vi "Save Console Logs.vi"(0 "Barcode":string, 11 "Error In":errorcluster) -> (15 "Error Out":errorcluster)   [LabVIEW 2021]
doc: "Creates a text file and dumps the console logs into it."
uses:
  Controls/Console Manager Functions.ctl
panel:
  # "Inputs"
  # "Outputs"
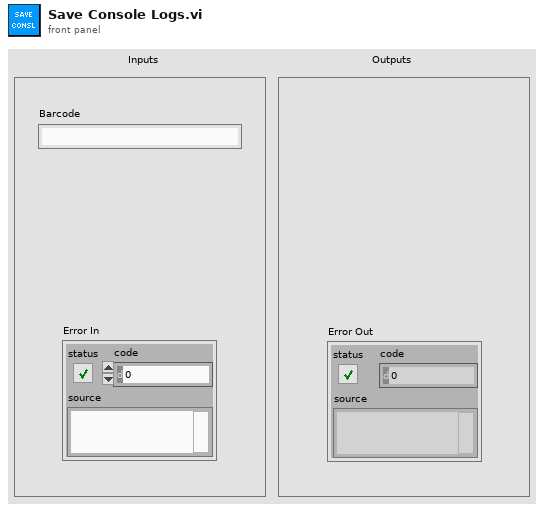
[diagram p1: front panel]
types:
  T1 = enum16{"open", "replace", "create", "open or create", "replace or create", "replace or create with confirmation"}
  T2 = typedef "Console Manager Functions.ctl" = enum16{"Init", "Add", "Get"}
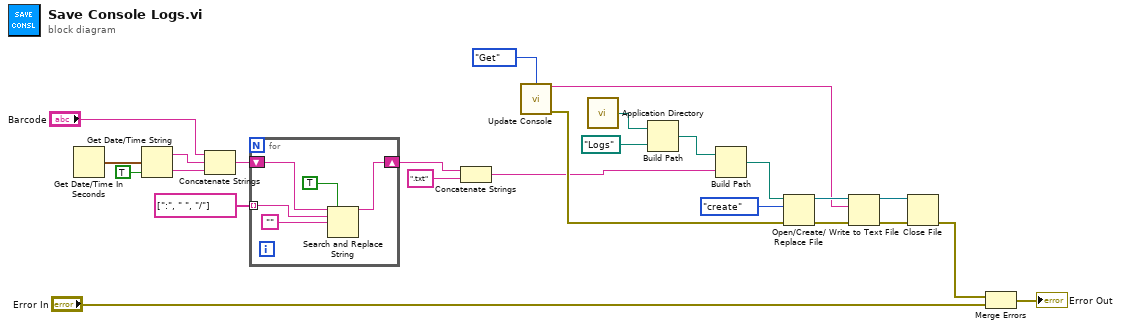
[diagram p0: block diagram]
diagram:
  n1 = Get Date/Time In Seconds() -> (seconds since 1Jan1904=w10:timestamp)
  n2 = Get Date/Time String(seconds (now)=w10, want seconds? (F)=TRUE) -> (date string=w7:string, time string=w8:string)  [unwired: 1 in]
  n3 = Concatenate Strings("Barcode", w7, w8) -> (w6:string)
  n4 = for {
    shift-right: [w27] -> w4
    shift-left: w6 -> [w29]
    tunnel: string[] [":", " ", "/"] ("search string") -> [w28] mode=indexing
    n5 = Search and Replace String(replace all?=TRUE ("replace all? (F)"), input string=w29, search string=w28, replace string="") -> (result string=w27:string)  [unwired: 4 in, 3 out]
  }
  n6 = Concatenate Strings(w4, ".txt" ("string")) -> (w2:string)
  n7 = call "Update Console.vi"("Function"=Console_Manager_Functions."Get") -> ("Existing String"=w11:string, "Error Out"=w12:errorcluster)  [unwired: 13 in]
  n8 = call <vilib>:"Application Directory.vi"() -> ("Application Directory"=w23:path)
  n9 = Build Path(base path=w23, name or relative path=path "Logs") -> (appended path=w21:path)
  n10 = Build Path(base path=w21, name or relative path=w2) -> (appended path=w17:path)
  n11 = Open/Create/Replace File(file path (use dialog)=w17, error in=w12, operation (0:open)=T1."create") -> (refnum out=w18:refnum<file>, error out=w19:errorcluster)  [unwired: 3 in, 1 out]
  n12 = Write to Text File(file (use dialog)=w18, text=w11, error in=w19) -> (refnum out=w20:refnum<file>, error out=w24:errorcluster)  [unwired: 1 in, 1 out]
  n13 = Close File(refnum=w20, error in=w24) -> (error out=w15:errorcluster)  [unwired: 1 out]
  n14 = Merge Errors(w15, "Error In") -> (→"Error Out":errorcluster)
